vi "FindAverageFRF_No Hammer.vi"(1 "Output":u16(ring)=1 items=["Accelerometer", "Accel (speed)", "Microphone", "Vibrometer"], 5 "Microphone Spectrum":cluster{dbl, "df":dbl, "FFT {X}":cdb[]}[](array[cluster])) -> (0 "Coherence":cluster{"x0":dbl, "df":dbl, dbl[]}(graph), 2 "Complex FRF":cluster{"t0":dbl, "dt":dbl, "Y":cdb[]}, 3 "Average FRF":cluster{"x0":dbl, "df":dbl, dbl[]}(graph))   [LabVIEW 2022 SP3]
panel:
  out "All runs (magnitude)":cluster{dbl, "df":dbl, "FFT {X}":dbl[]}[](graph)
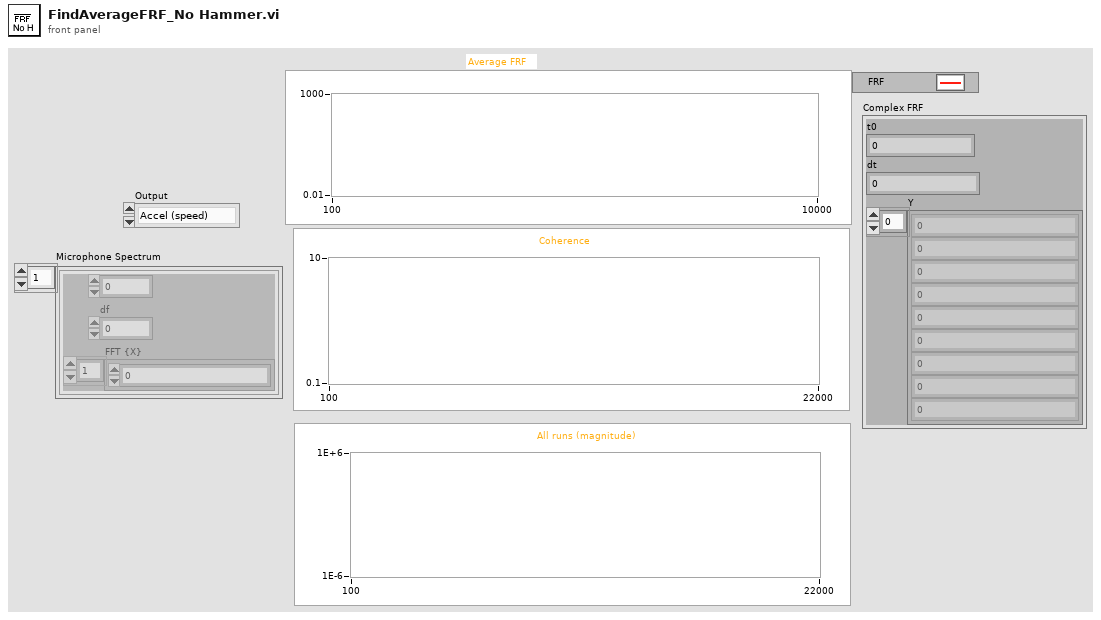
[diagram p1: front panel]
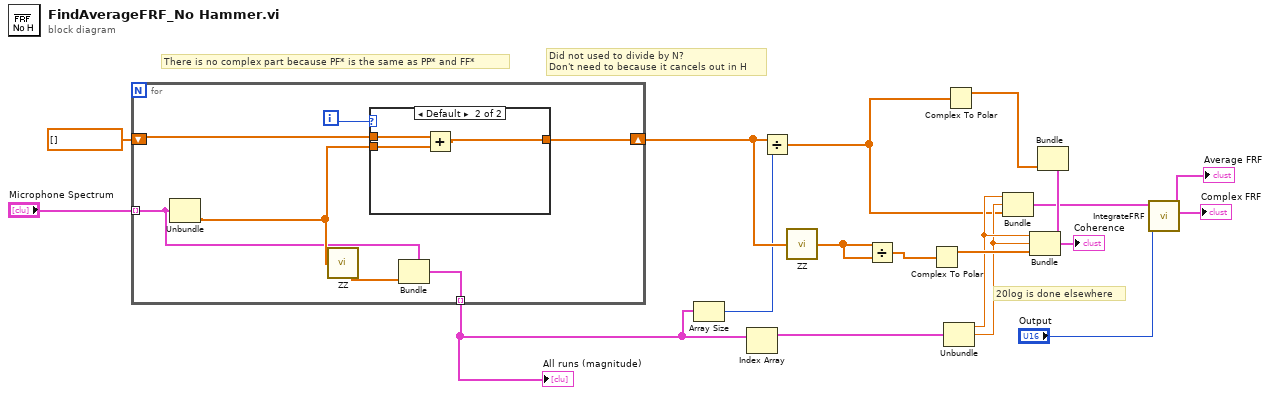
[diagram p0: block diagram]
diagram:
  # "There is no complex part because PF* is the same as PP* and FF*"
  # "20log is done elsewhere"
  # "Did not used to divide by N?\nDon't need to because it cancels out in H"
  n1 = for {
    shift-right: [w24] -> w15
    shift-left: cdb[] [] ("PF*") -> [w25]
    tunnel: "Microphone Spectrum" -> [w20] mode=indexing
    tunnel: [w19] -> w5 mode=indexing
    i -> [w23]
    n2 = Unbundle(w20) -> ("FFT {X}"=w22:cdb[])  [unwired: 2 out]
    n3 = call "ZZ.vi"("P"=w22) -> ("PP*"=w21:dbl[])
    n4 = case shown="Default" w23 {
      tunnel: w22 -> [w26 w29]
      tunnel: w25 -> [_ w28]
      tunnel: [w26 w27] -> w24
      frame 0 {
      }
      frame Default {
        n5 = Add(x=w28, y=w29) -> (x+y=w27:cdb[])
      }
    }
    n6 = Bundle(cluster=w20, "FFT {X}"=w21) -> (w19:cluster{dbl, "df":dbl, "FFT {X}":cdb[]})  [unwired: 2 in]
  }
  "All runs (magnitude)" <- w5
  n7 = Array Size(array=w5) -> (size(s)=w8:i32)
  n8 = Index Array(array=w5) -> (element=w14:cluster{dbl, "df":dbl, "FFT {X}":cdb[]})  [unwired: 1 in]
  n9 = Divide(x=w15, y=w8) -> (x/y=w11:cdb[])
  n10 = call "ZZ.vi"("P"=w15) -> ("PP*"=w9:dbl[])
  n11 = Divide(x=w9, y=w9) -> (x/y=w18:dbl[])
  n12 = Complex To Polar(r * e^(i*theta)=w18) -> (r=w16:dbl[])  [unwired: 1 out]
  n13 = Unbundle(w14) -> (w13:dbl, "df"=w12:dbl)  [unwired: 1 out]
  n14 = Complex To Polar(r * e^(i*theta)=w11) -> (r=w10:dbl[])  [unwired: 1 out]
  n15 = Bundle(w13, "df"=w12, w11) -> (w3:cluster{dbl, "df":dbl, cdb[]})  [unwired: 1 in]
  n16 = Bundle(w13, "df"=w12, w16) -> (w7:cluster{dbl, "df":dbl, dbl[]})  [unwired: 1 in]
  "Coherence" <- w7
  n17 = Bundle(cluster=w7, w10) -> ()  [unwired: 2 in, 1 out]
  n18 = call "IntegrateFRF.vi"("Output"="Output", "Complex FRF"=w3) -> ("Complex FRF out"=→"Complex FRF":cluster{"t0":dbl, "dt":dbl, "Y":cdb[]}, "FRF out"=→"Average FRF":cluster{"t0":dbl, "dt":dbl, dbl[]})  [unwired: 8 in]
